vi "Read Key Value Boolean.vi"(7 "Section Name":string, 8 "error in (no error)":errorcluster, 9 "Default":bool, 10 "Key Name":string, 11 "Ini-File in":refnum<class "Ini-File.lvclass">) -> (0 "error out":errorcluster, 1 "Value":bool, 2 "found":bool, 3 "Ini-File out":refnum<class "Ini-File.lvclass">)   [LabVIEW 2015, in "Configuration.lvlib" / "Ini-File.lvclass"]
doc: "Read boolean value."
uses:
  Ini-File.lvclass
  Ini-File.lvclass/Ini-File.ctl
  <vilib>/Utility/config.llb/Read Key (Boolean).vi
  <vilib>/Utility/config.llb/NI_LVConfig.lvlib
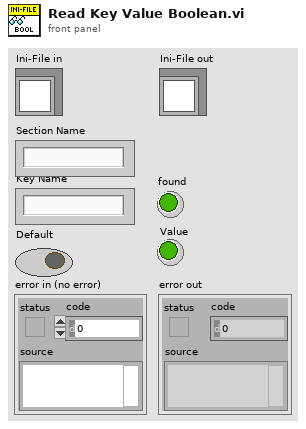
[diagram p1: front panel]
types:
  T1 = typedef "NI_LVConfig.lvlib/Config Data RefNum.ctl" = refnum<k1>
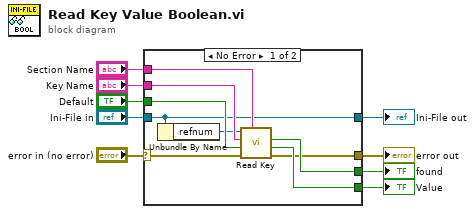
[diagram p0: block diagram]
diagram:
  n1 = case shown="No Error" "error in (no error)" {
    selector: "error in (no error)" -> [w10 w19]
    tunnel: "Ini-File in" -> [w12 w20]
    tunnel: "Key Name" -> [w18 _]
    tunnel: "Section Name" -> [w17 _]
    tunnel: "Default" -> [w16 _]
    tunnel: [w13 w19] -> w5
    tunnel: [w14 _] -> w4
    tunnel: [w15 _] -> w3
    tunnel: [w12 w20] -> w1
    frame No Error {
      n2 = Unbundle By Name(w12) -> ("refnum"=w11:T1)
      n3 = call-poly <vilib>:"Read Key.vi"("section"=w17, "error in (no error)"=w10, "default value"=w16, "key"=w18, "refnum"=w11) -> ("error out"=w13:errorcluster, "value"=w14:bool, "found?"=w15:bool)  [unwired: 3 in, 1 out]
    }
    frame Error {
    }
  }
  "error out" <- w5
  "Ini-File out" <- w1
  "Value" <- w4
  "found" <- w3
